vi "Create folder path if needed from file path.vi"(8 "error in":errorcluster, 11 "String file path":string) -> (0 "error out":errorcluster, 2 "file exists?":bool, 3 "File Path":path)   [LabVIEW 2013]
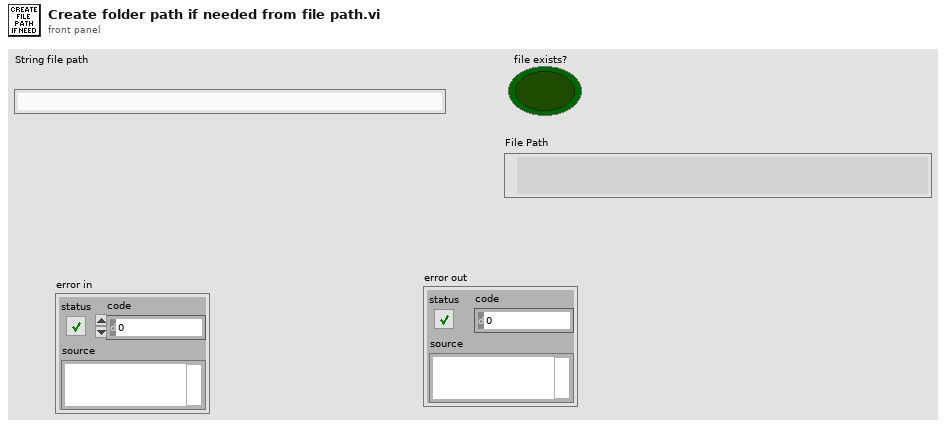
[diagram p1: front panel]
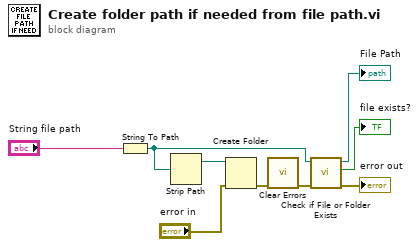
[diagram p0: block diagram]
diagram:
  n1 = String To Path(string="String file path") -> (path=w2:path)
  n2 = Strip Path(path=w2) -> (stripped path=w9:path)  [unwired: 1 out]
  n3 = Create Folder(path (use dialog)=w9, error in="error in") -> (error out=w8:errorcluster)  [unwired: 1 in, 2 out]
  n4 = call <vilib>:"Clear Errors.vi"("error in (no error)"=w8) -> ("error out"=w5:errorcluster)  [unwired: 6 in]
  n5 = call <vilib>:"Check if File or Folder Exists.vi"("error in (no error)"=w5, "path"=w2) -> ("error out"=→"error out":errorcluster, "file or folder exists?"=→"file exists?":bool, "dup path"=→"File Path":path)  [unwired: 7 in]
